vi "GE 5565PIORC.DMA.Scatter-Gather.Set Descriptor Params.vi"(8 "error in (no error)":errorcluster, 9 "descriptor params":T1 {"data ptr (lower)" format="%.0x"; "data ptr (upper)" format="%.0x"; "data size" format="%.0x"; "next descriptor ptr" format="%.0x"}, 10 "descriptor ptr":u32 format="%08x", 11 "GE 5565PIORC in":refnum<class "GE 5565PIORC.lvclass">) -> (0 "error out":errorcluster, 3 "GE 5565PIORC out":refnum<class "GE 5565PIORC.lvclass">)   [LabVIEW 2017, in "GE 5565PIORC.lvclass"]
doc: "Writes the <B>descriptor params</B> to PCI Memory space at the location specified by <B>descriptor ptr</B>."
uses:
  GE 5565PIORC.lvclass
  Typedefs/GE 5565PIORC.Typedef.DMA Block Descriptor Params.ctl
  GE 5565PIORC.lvclass/GE 5565PIORC.ctl
  <vilib>/Instr/_visa.llb/VISA Register Access Address Space.ctl
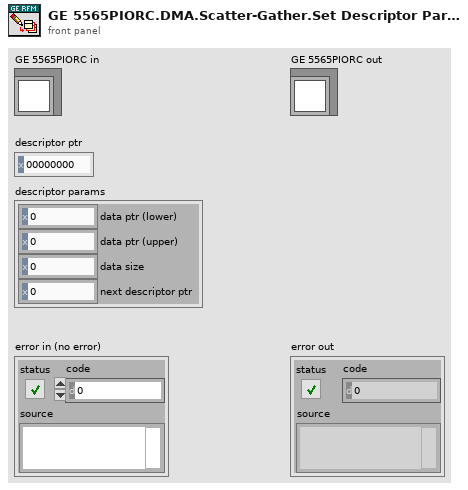
[diagram p1: front panel]
types:
  T1 = typedef "GE 5565PIORC.lvclass/GE 5565PIORC.Typedef.DMA Block Descriptor Params.ctl" = cluster{"data ptr (lower)":u32, "data ptr (upper)":u32, "data size":u32, "next descriptor ptr":u32}
  T2 = typedef "VISA Register Access Address Space.ctl" = u16
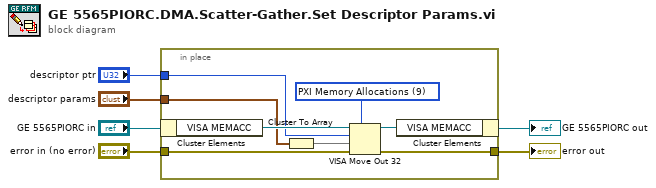
[diagram p0: block diagram]
diagram:
  n1 = in-place {
    in-place-border: "error in (no error)" -> [w14]
    in-place-border: [w11] -> w4
    in-place-border: "descriptor params" -> [w9]
    in-place-border: "descriptor ptr" -> [w7]
    w10 = T2 9 items=["VXI/VME A16"=1, "VXI/VME A24"=2, "VXI/VME A32"=3, "VXI/VME A64"=4, "PXI Memory Allocations"=9, "PXI Configuration"=10, "PXI BAR0"=11, "PXI BAR1"=12, "PXI BAR2"=13, "PXI BAR3"=14, "PXI BAR4"=15, "PXI BAR5"=16] ("Address Space")
    n2 = in-place-cluster #1("GE 5565PIORC in") -> ("VISA MEMACC"=w13:refnum<visa-resource-name>)
    n3 = Cluster To Array(cluster=w9) -> (array=w8:u32[])
    n4 = VISA Move Out 32(7:w10, 8:w14, 9:w8, 10:w7, 11:w13) -> (0:w11:errorcluster, 3:w12:refnum<visa-resource-name>)
    n5 = in-place-cluster #1("VISA MEMACC"=w12) -> (→"GE 5565PIORC out":refnum<class "GE 5565PIORC.lvclass">)
  }
  "error out" <- w4
